vi "EIP Get Tag Info.vi"(8 "error in":errorcluster, 10 "Specified Channel Ref List":T1[](array[typedef]) format="%.0x", 11 "Item Ref in":T1 format="%.0x") -> (0 "error out":errorcluster, 2 "Tag Data":T2[](array[typedef]) {"Device Reference" format="%.0x"}, 3 "Item Ref out":T1 format="%.0x")   [LabVIEW 2023, in "Ethernet IP Custom Device Custom Device.lvlib"]
uses:
  Ethernet IP Custom Device Custom Device.lvlib
  <vilib>/NI VeriStand/Custom Device API/Custom Device Item Ref.ctl
  EIP Tag Information.ctl
  <vilib>/NI VeriStand/Custom Device API/Custom Device Item Info.ctl
  L5K Data Types.ctl
  EIP Message Type.ctl
  EIP Attribute Info.ctl
  Ethernet IP Global Strings.vi
  <vilib>/NI VeriStand/Custom Device API/Get Item Property (U16).vi
  <vilib>/NI VeriStand/Custom Device API/Get Item Property (String).vi
  <vilib>/NI VeriStand/Custom Device API/Get Item Property (Variant).vi
  <vilib>/NI VeriStand/Custom Device API/Custom Device API.lvlib
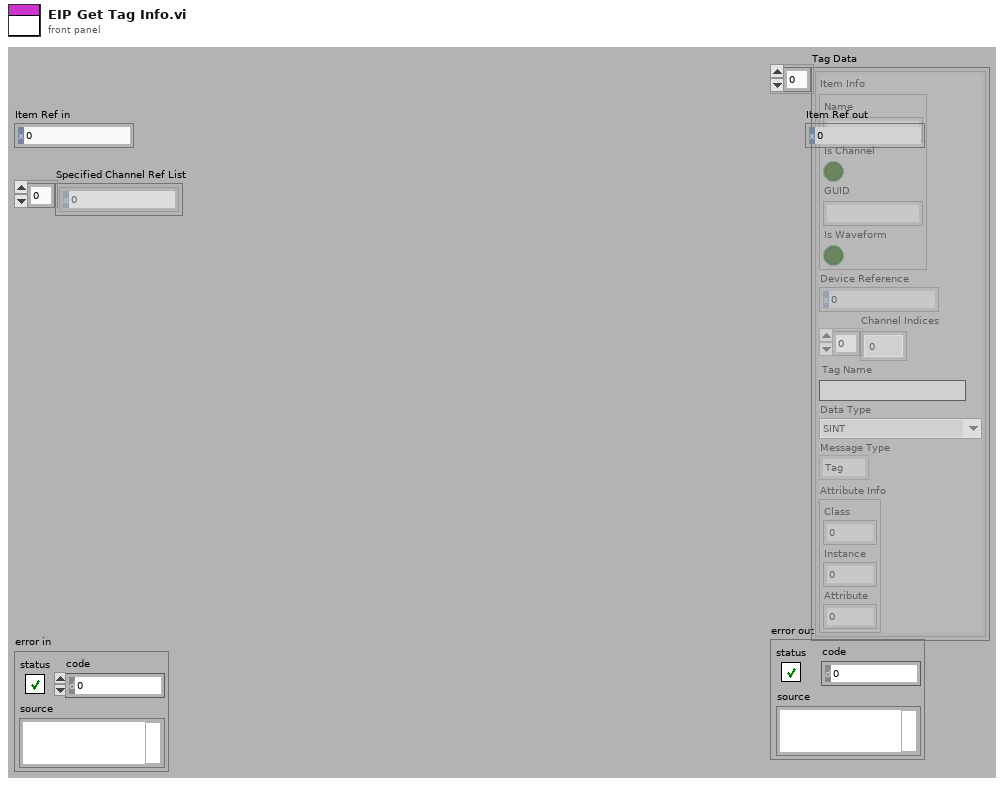
[diagram p1: front panel]
types:
  T1 = typedef "Custom Device API.lvlib/Custom Device Item Ref.ctl" = u64
  T2 = typedef "Ethernet IP Custom Device Custom Device.lvlib/EIP Tag Information.ctl" = cluster{"Item Info":T3, "Device Reference":T1, "Channel Indices":i32[], "Tag Name":string, "Data Type":T4, "Message Type":T5, "Attribute Info":T6}
  T3 = typedef "Custom Device API.lvlib/Custom Device Item Info.ctl" = cluster{"Name":string, "Is Channel":bool, "GUID":string, "Is Waveform":bool}
  T4 = typedef "Ethernet IP Custom Device Custom Device.lvlib/L5K Data Types.ctl" = enum16{"SINT", "INT", "DINT", "REAL", "BOOL"}
  T5 = typedef "EIP Message Type.ctl" = enum16{"Tag", "Attribute"}
  T6 = typedef "EIP Attribute Info.ctl" = cluster{"Class":i32, "Instance":u32, "Attribute":i32}
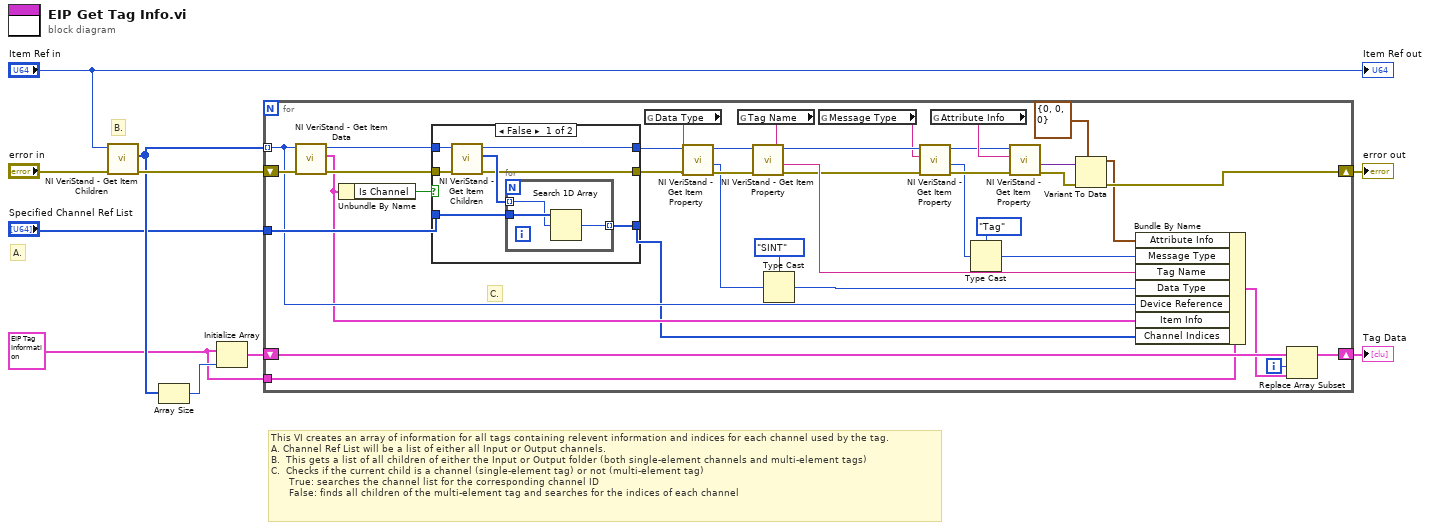
[diagram p0: block diagram]
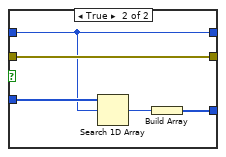
[diagram p2: hidden frame]
diagram:
  w3 = T2 {"Item Info"={"Name"="", "Is Channel"=FALSE, "GUID"="", "Is Waveform"=FALSE}, "Device Reference"=0, "Channel Indices"=[], "Tag Name"="", "Data Type"=enum."SINT", "Message Type"=enum."Tag", "Attribute Info"={"Class"=0, "Instance"=0, "Attribute"=0}} ("EIP Tag Information")
  # "B."
  # "A."
  # "This VI creates an array of information for all tags containing relevent information and indices for each channel used by the tag.\nA. Channel Ref List will be a list of either all Input or Output channels.\nB.  This gets a list of all children of either the Input or Output folder (both single-element channels and multi-element tags)\nC.  Checks if the current child is a channel (single-element tag) or not (multi-element tag)\n      True: searches the channel list for the corresponding channel ID \n      False: finds all children of the multi-element tag and searches for the indices of each channel"
  n1 = call <vilib>:"NI VeriStand - Get Item Children.vi"("error in (no error)"="error in", "Item Ref in"="Item Ref in") -> ("error out"=w10:errorcluster, "Child Refs"=w8:T1[])  [unwired: 6 in, 2 out]
  n2 = Array Size(array=w8) -> (size(s)=w7:i32)
  n3 = Initialize Array(w3, w7) -> (w6:T2[])
  n4 = for {
    tunnel: w8 -> [w39] mode=indexing
    tunnel: "Specified Channel Ref List" -> [w45]
    shift-right: [w12] -> w9
    shift-left: w10 -> [w44]
    shift-right: [w41] -> w2
    shift-left: w6 -> [w42]
    tunnel: w3 -> [w40]
    i -> [w35]
    # "C."
    n5 = call <vilib>:"NI VeriStand - Get Item Data.vi"("error in (no error)"=w44, "Item Ref in"=w39) -> ("error out"=w43:errorcluster, "Item Info"=w38:T3, "Item Ref out"=w46:T1)  [unwired: 6 in, 1 out]
    n6 = Unbundle By Name(w38) -> ("Is Channel"=w47:bool)
    n7 = case shown="False" w47 {
      tunnel: w46 -> [w54 w58]
      tunnel: w45 -> [w52 w62]
      tunnel: w43 -> [w51 w61]
      tunnel: [w49 w61] -> w33
      tunnel: [w50 w59] -> w37
      tunnel: [w48 w58] -> w32
      frame False {
        n8 = call <vilib>:"NI VeriStand - Get Item Children.vi"("error in (no error)"=w51, "Item Ref in"=w54) -> ("error out"=w49:errorcluster, "Child Refs"=w53:T1[], "Item Ref out"=w48:T1)  [unwired: 6 in, 1 out]
        n9 = for {
          tunnel: w53 -> [w56] mode=indexing
          tunnel: w52 -> [w57]
          tunnel: [w55] -> w50 mode=indexing
          n10 = Search 1D Array(1D array=w57, element=w56) -> (index of element=w55:i32)  [unwired: 1 in]
        }
      }
      frame True {
        n11 = Search 1D Array(1D array=w62, element=w58) -> (index of element=w60:i32)  [unwired: 1 in]
        n12 = Build Array(w60) -> (w59:i32[])
      }
    }
    n13 = global read "Ethernet IP Global Strings.vi" "Data Type"() -> (w26:string)
    n14 = call-poly <vilib>:"NI VeriStand - Get Item Property.vi"("error in (no error)"=w33, "Property Name"=w26, "Item Ref in"=w32) -> ("error out"=w34:errorcluster, "Value"=w28:u16, "Item Ref out"=w31:T1)  [unwired: 5 in, 1 out]
    n15 = global read "Ethernet IP Global Strings.vi" "Tag Name"() -> (w25:string)
    n16 = call-poly <vilib>:"NI VeriStand - Get Item Property.vi"("error in (no error)"=w34, "Property Name"=w25, "Item Ref in"=w31) -> ("error out"=w22:errorcluster, "Value"=w30:string, "Item Ref out"=w23:T1)  [unwired: 5 in, 1 out]
    n17 = Type Cast(type=L5K_Data_Types."SINT" ("Data Type"), x=w28) -> (*(type *) &x=w29:T4)
    n18 = global read "Ethernet IP Global Strings.vi" "Message Type"() -> (w21:string)
    n19 = call-poly <vilib>:"NI VeriStand - Get Item Property.vi"("error in (no error)"=w22, "Property Name"=w21, "Item Ref in"=w23) -> ("error out"=w24:errorcluster, "Value"=w19:u16, "Item Ref out"=w16:T1)  [unwired: 5 in, 1 out]
    n20 = global read "Ethernet IP Global Strings.vi" "Attribute Info"() -> (w17:string)
    n21 = Type Cast(type=EIP_Message_Type."Tag" ("Message Type"), x=w19) -> (*(type *) &x=w18:T5)
    n22 = call-poly <vilib>:"NI VeriStand - Get Item Property.vi"("error in (no error)"=w24, "Property Name"=w17, "Item Ref in"=w16) -> ("error out"=w13:errorcluster, "Value"=w14:variant)  [unwired: 5 in, 2 out]
    n23 = Variant To Data(error in=w13, type=T6 {"Class"=0, "Instance"=0, "Attribute"=0} ("Attribute Info"), Variant=w14) -> (data=w11:T6, error out=w12:errorcluster)
    n24 = Bundle By Name(cluster=w40, "Attribute Info"=w11, "Message Type"=w18, "Tag Name"=w30, "Data Type"=w29, "Device Reference"=w39, "Item Info"=w38, "Channel Indices"=w37) -> (w36:T2)
    n25 = Replace Array Subset(array=w42, new element=w36, index=w35) -> (w41:T2[])
  }
  "error out" <- w9
  "Tag Data" <- w2
  "Item Ref out" <- "Item Ref in"
